vi "Visualize Manhattan Distances.vi"(10 "Range":i32[](array[numeric]), 11 "Coordinates":i32[][](array[numeric])) -> (3 "Manhattan Distances":i32[][][](array[numeric]))   [LabVIEW 2019]
doc: "Given a range of the min and max coordinate values, and the coordinates, output a 3D array where each page represents a coordinate, and the manhattan distance values are displayed at every coordinate pair in the range."
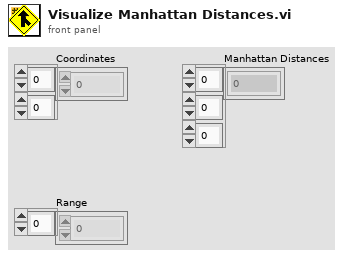
[diagram p1: front panel]
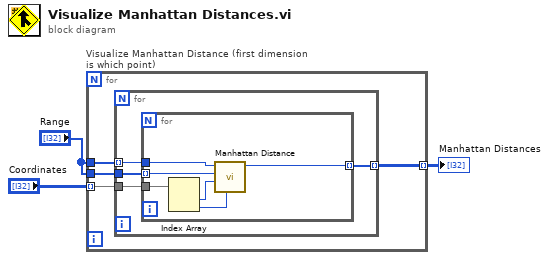
[diagram p0: block diagram]
diagram:
  n1 = for "Visualize Manhattan Distance (first dimension is which point)" {
    tunnel: "Range" -> [w6]
    tunnel: "Range" -> [w7]
    tunnel: "Coordinates" -> [w5] mode=indexing
    tunnel: [w4] -> w1 mode=indexing
    n2 = for {
      tunnel: w7 -> [w10]
      tunnel: w6 -> [w9] mode=indexing
      tunnel: w5 -> [w11]
      tunnel: [w8] -> w4 mode=indexing
      n3 = for {
        tunnel: w11 -> [w17]
        tunnel: w10 -> [w13] mode=indexing
        tunnel: w9 -> [w14]
        tunnel: [w12] -> w8 mode=indexing
        n4 = Index Array(array=w17) -> (element #1=w16:i32, element #2=w15:i32)  [unwired: 2 in]
        n5 = call "Manhattan Distance.vi"("y 2"=w15, "x 2"=w16, "x"=w13, "y"=w14) -> ("Manhattan Distance"=w12:i32)  [unwired: 7 in]
      }
    }
  }
  "Manhattan Distances" <- w1
